vi "Find GALVO SPOT (SubVI).vi"(0 "REF In":refnum<k21>, 7 "Stopped?":refnum<vi>, 8 "GALVO #":T1(ring), 10 "IR SPOT (Target)":cluster{"X":i32, "Y":i32}, 12 "GALVO Input Voltage (V)":refnum<vi>, 14 "IR SPOT (Measured)":refnum<vi>, 16 "X Reverse":bool, 18 "Y Reverse":bool) -> (20 "REF Out":refnum<k21>)   [LabVIEW 2017]
uses:
  <vilib>/DAQmx/write.llb/DAQmx Write (Analog 1D DBL NChan 1Samp).vi
  <vilib>/DAQmx/miscellaneous.llb/DAQmx Fill In Error Info.vi
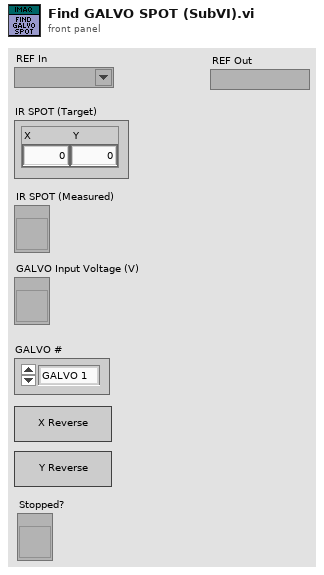
[diagram p1: front panel]
types:
  T1 = enum16{"GALVO 1", "GALVO 2", "GALVO 3", "GALVO 4"}
  T2 = cluster{"GALVO 1":cluster{"X":dbl, "Y ":dbl}, "GALVO 2":cluster{"X":dbl, "Y ":dbl}, "GALVO 3":cluster{"X":dbl, "Y ":dbl}, "GALVO 4":cluster{"X":dbl, "Y ":dbl}}
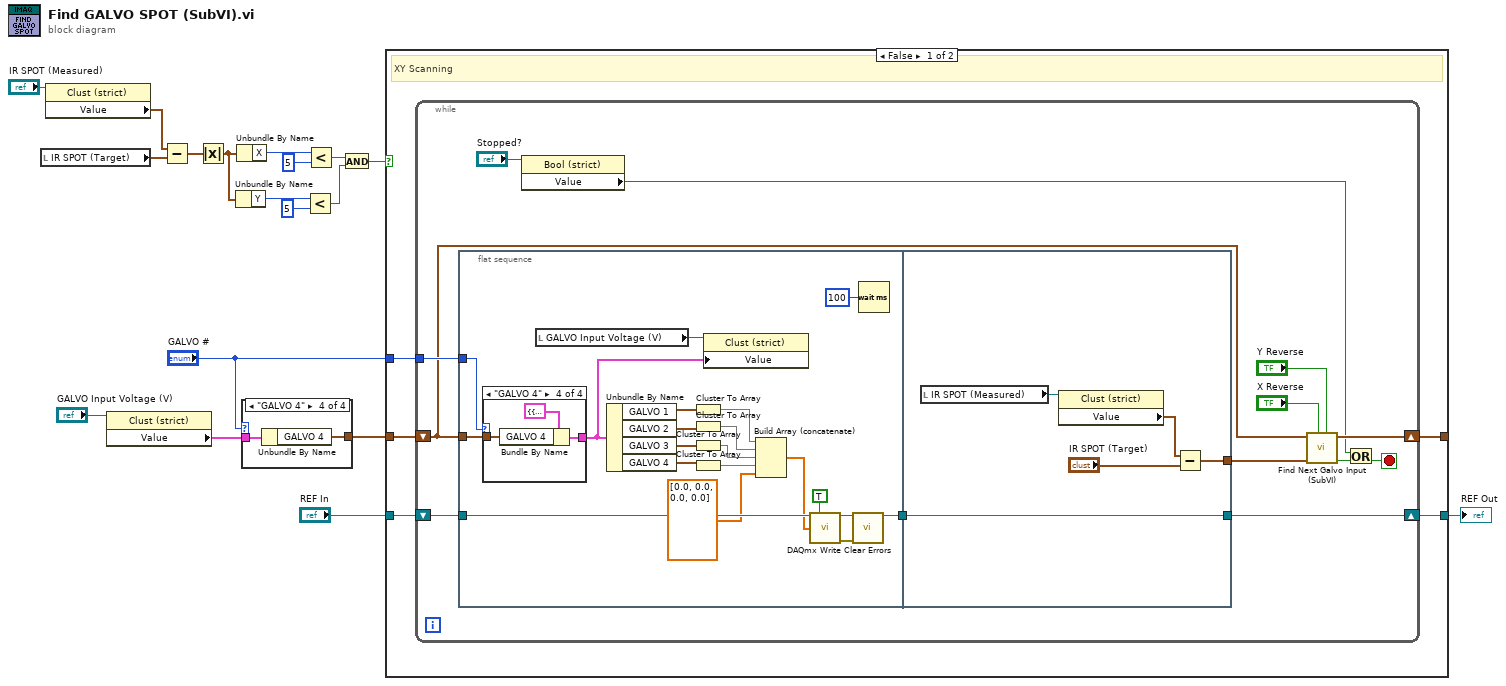
[diagram p0: block diagram]
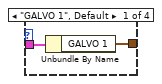
[diagram p2: hidden frame]
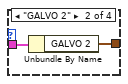
[diagram p3: hidden frame]
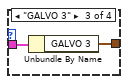
[diagram p4: hidden frame]
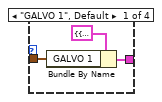
[diagram p5: hidden frame]
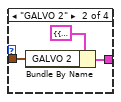
[diagram p6: hidden frame]
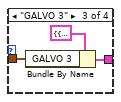
[diagram p7: hidden frame]
diagram:
  n1 = local read "IR SPOT (Target)"() -> (w14:cluster{"X":i32, "Y":i32})
  n2 = property class="Clust (strict)"(reference="IR SPOT (Measured)") -> ("Value"=w15:cluster{"X":i32, "Y":i32})  [unwired: 1 in, 2 out]
  n3 = property class="Clust (strict)"(reference="GALVO Input Voltage (V)") -> ("Value"=w9:T2)  [unwired: 1 in, 2 out]
  n4 = Subtract(x=w15, y=w14) -> (x-y=w18:cluster{"X":i32, "Y":i32})
  n5 = Absolute Value(x=w18) -> (abs(x)=w4:cluster{"X":i32, "Y":i32})
  n6 = Unbundle By Name(w4) -> ("Y"=w5:i32)
  n7 = Unbundle By Name(w4) -> ("X"=w16:i32)
  n8 = case shown="\"GALVO 4\"" "GALVO #" {
    tunnel: w9 -> [w20 w22 w24 w26]
    tunnel: [w19 w21 w23 w25] -> w8
    frame "GALVO 1", Default {
      n9 = Unbundle By Name(w20) -> ("GALVO 1"=w19:cluster{"X":dbl, "Y ":dbl})
    }
    frame "GALVO 2" {
      n10 = Unbundle By Name(w22) -> ("GALVO 2"=w21:cluster{"X":dbl, "Y ":dbl})
    }
    frame "GALVO 3" {
      n11 = Unbundle By Name(w24) -> ("GALVO 3"=w23:cluster{"X":dbl, "Y ":dbl})
    }
    frame "GALVO 4" {
      n12 = Unbundle By Name(w26) -> ("GALVO 4"=w25:cluster{"X":dbl, "Y ":dbl})
    }
  }
  n13 = Less?(x=w5, y=5) -> (x < y?=w2:bool)
  n14 = Less?(x=w16, y=5) -> (x < y?=w7:bool)
  n15 = And(x=w7, y=w2) -> (x .and. y?=w3:bool)
  n16 = case shown="False" w3 {
    tunnel: "REF In" -> [w31 w82]
    tunnel: [w30 w82] -> w12
    tunnel: w8 -> [w29 w81]
    tunnel: [w28 w81] -> _
    tunnel: "GALVO #" -> [w27 _]
    frame False {
      # "XY Scanning"
      n17 = while {
        shift-right: [w43] -> w30
        shift-left: w31 -> [w44]
        shift-right: [w42] -> w28
        shift-left: w29 -> [w35]
        tunnel: w27 -> [w41]
        stop <- w33 stop-if-true
        n18 = flat-sequence {
          tunnel: w44 -> [w63]
          tunnel: w35 -> [w61]
          tunnel: w41 -> [w60]
          tunnel: [w62] -> w40
          tunnel: [w80] -> w43
          tunnel: w40 -> [w80]
          tunnel: [w76] -> w36
          frame #0 {
            n19 = case shown="\"GALVO 4\"" w60 {
              tunnel: w61 -> [w65 w68 w71 w74]
              tunnel: [w64 w67 w70 w73] -> w47
              frame "GALVO 1", Default {
                n20 = Bundle By Name(cluster=T2 {"GALVO 1"={"X"=-1.0, "Y "=1.0}, "GALVO 2"={"X"=0.0, "Y "=0.0}, "GALVO 3"={"X"=0.0, "Y "=0.0}, "GALVO 4"={"X"=0.0, "Y "=0.0}} ("GALVO Input Voltage (V)"), "GALVO 1"=w65) -> (w64:T2)
              }
              frame "GALVO 2" {
                n21 = Bundle By Name(cluster=T2 {"GALVO 1"={"X"=-1.0, "Y "=1.0}, "GALVO 2"={"X"=0.0, "Y "=0.0}, "GALVO 3"={"X"=0.0, "Y "=0.0}, "GALVO 4"={"X"=0.0, "Y "=0.0}} ("GALVO Input Voltage (V)"), "GALVO 2"=w68) -> (w67:T2)
              }
              frame "GALVO 3" {
                n22 = Bundle By Name(cluster=T2 {"GALVO 1"={"X"=-1.0, "Y "=1.0}, "GALVO 2"={"X"=0.0, "Y "=0.0}, "GALVO 3"={"X"=0.0, "Y "=0.0}, "GALVO 4"={"X"=0.0, "Y "=0.0}} ("GALVO Input Voltage (V)"), "GALVO 3"=w71) -> (w70:T2)
              }
              frame "GALVO 4" {
                n23 = Bundle By Name(cluster=T2 {"GALVO 1"={"X"=-1.0, "Y "=1.0}, "GALVO 2"={"X"=0.0, "Y "=0.0}, "GALVO 3"={"X"=0.0, "Y "=0.0}, "GALVO 4"={"X"=0.0, "Y "=0.0}} ("GALVO Input Voltage (V)"), "GALVO 4"=w74) -> (w73:T2)
              }
            }
            n24 = local read "GALVO Input Voltage (V)"() -> (w46:refnum<vi>)
            n25 = Unbundle By Name(w47) -> ("GALVO 1"=w51:cluster{"X":dbl, "Y ":dbl}, "GALVO 2"=w52:cluster{"X":dbl, "Y ":dbl}, "GALVO 3"=w53:cluster{"X":dbl, "Y ":dbl}, "GALVO 4"=w54:cluster{"X":dbl, "Y ":dbl})
            n26 = Cluster To Array(cluster=w51) -> (array=w55:dbl[])
            n27 = Cluster To Array(cluster=w52) -> (array=w56:dbl[])
            n28 = Cluster To Array(cluster=w53) -> (array=w57:dbl[])
            n29 = Cluster To Array(cluster=w54) -> (array=w58:dbl[])
            n30 = property class="Clust (strict)"(reference=w46, "Value"=w47) -> ()  [unwired: 1 in, 2 out]
            n31 = Build Array (concatenate)(w55, w56, w57, w58, dbl[] [0.0, 0.0, 0.0, 0.0] ("array")) -> (w59:dbl[])
            n32 = call-poly <vilib>:"DAQmx Write.vi"("task/channels in"=w63, "auto start"=TRUE, "data"=w59) -> ("task out"=w62:refnum<k21>, "error out"=w50:errorcluster)  [unwired: 10 in, 1 out]
            n33 = call <vilib>:"Clear Errors.vi"("error in (no error)"=w50) -> ()  [unwired: 5 in, 2 out]
            n34 = Wait (ms)(milliseconds to wait=u32 100) -> ()  [unwired: 1 out]
          }
          frame #1 {
            n35 = local read "IR SPOT (Measured)"() -> (w79:refnum<vi>)
            n36 = property class="Clust (strict)"(reference=w79) -> ("Value"=w77:cluster{"X":i32, "Y":i32})  [unwired: 1 in, 2 out]
            n37 = Subtract(x=w77, y="IR SPOT (Target)") -> (x-y=w76:cluster{"X":i32, "Y":i32})
          }
        }
        n38 = property class="Bool (strict)"(reference="Stopped?") -> ("Value"=w32:bool)  [unwired: 1 in, 2 out]
        n39 = call "Find Next Galvo Input (SubVI).vi"("Y Reverse"="Y Reverse", "X Reverse"="X Reverse", "Deviation"=w36, "Current GALVO Voltage"=w35) -> ("Target Spot Reached?"=w39:bool, "Next GALVO Volage"=w42:cluster{"X":dbl, "Y ":dbl})  [unwired: 6 in]
        n40 = Or(x=w32, y=w39) -> (x .or. y?=w33:bool)
      }
    }
    frame True {
    }
  }
  "REF Out" <- w12
